vi "StartSpinningDisc.vi"(8 "error in (no error)":errorcluster) -> (0 "error out":errorcluster)   [LabVIEW 2015]
panel:
  out "return count":u32
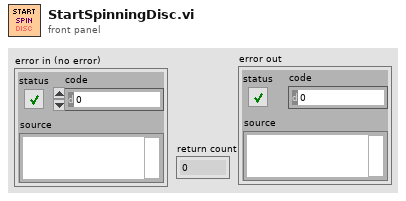
[diagram p1: front panel]
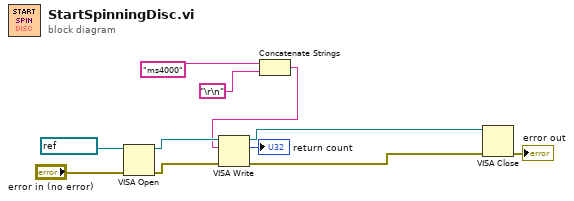
[diagram p0: block diagram]
diagram:
  n1 = VISA Open(error in (no error)="error in (no error)", VISA resource name=refnum<visa-resource-name> "COM1") -> (VISA resource name=w8:refnum<visa-resource-name>, error out=w9:errorcluster)  [unwired: 3 in]
  n2 = Concatenate Strings("ms4000", "\r\n") -> (w6:string)
  n3 = VISA Write(VISA resource name=w8, write buffer=w6, error in (no error)=w9) -> (VISA resource name out=w4:refnum<visa-resource-name>, return count=→"return count":u32, error out=w3:errorcluster)
  n4 = VISA Close(VISA resource name=w4, error in (no error)=w3) -> (error out=→"error out":errorcluster)
